vi "publish -- lorentzian.vi"(7 "publisher action":T3, 9 "lorentzian IN":T1={"A (VHz)"=1.0, "f (Hz)"=1000.0, "G (Hz)"=3.0, "phi(rad)"=0.0, "Q"=300.0, "Norm  Ampl"=nan, "bg (V)"=0.0+0.0i, "4corners"={"z (-pi/2)"=9.277908004825974e-07+0.0007240755403629966i, "z(inf)"=2.6527949823343002e-05+0.0007477540585896028i, "z (pi/2)"=2.8494315967368497e-06+0.0007733542176124632i, "z center"=1.8886111986097237e-06+0.0007487148789877299i, "z(0)"=-2.2750727426123552e-05+0.000749675699385857i, "radius"=2.4658065287076567e-05}} {"bg (V)" format="%#_3p"; "Q" format="%#_4p"; "phi(rad)" format="%#_3p"; "G (Hz)" format="%#_4p"; "f (Hz)" format="%#_6p"; "A (VHz)" format="%#_3p"}) -> (1 "lorentzian OUT":T1={"A (VHz)"=1.0, "f (Hz)"=1000.0, "G (Hz)"=3.0, "phi(rad)"=0.0, "Q"=300.0, "Norm  Ampl"=nan, "bg (V)"=0.0+0.0i, "4corners"={"z (-pi/2)"=9.277908004825974e-07+0.0007240755403629966i, "z(inf)"=2.6527949823343002e-05+0.0007477540585896028i, "z (pi/2)"=2.8494315967368497e-06+0.0007733542176124632i, "z center"=1.8886111986097237e-06+0.0007487148789877299i, "z(0)"=-2.2750727426123552e-05+0.000749675699385857i, "radius"=2.4658065287076567e-05}} {"bg (V)" format="%#_3p"; "Q" format="%#_4p"; "phi(rad)" format="%#_3p"; "G (Hz)" format="%#_4p"; "f (Hz)" format="%#_6p"; "A (VHz)" format="%#_3p"})   [LabVIEW 2020]
uses:
  publisher action.ctl
  lorentzian.ctl
  circle corners.ctl
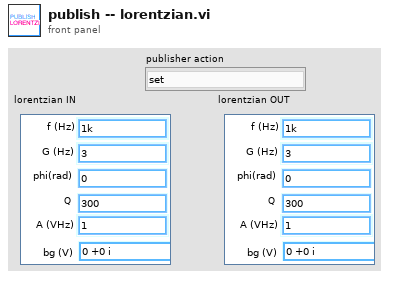
[diagram p1: front panel]
types:
  T1 = typedef "lorentzian.ctl" = cluster{"A (VHz)":dbl, "f (Hz)":dbl, "G (Hz)":dbl, "phi(rad)":dbl, "Q":dbl, "Norm  Ampl":dbl, "bg (V)":cdb, "4corners":T2}
  T2 = typedef "circle corners.ctl" = cluster{"z (-pi/2)":cdb, "z(inf)":cdb, "z (pi/2)":cdb, "z center":cdb, "z(0)":cdb, "radius":dbl}
  T3 = typedef "publisher action.ctl" = enum16{"set", "get", "init", "check"}
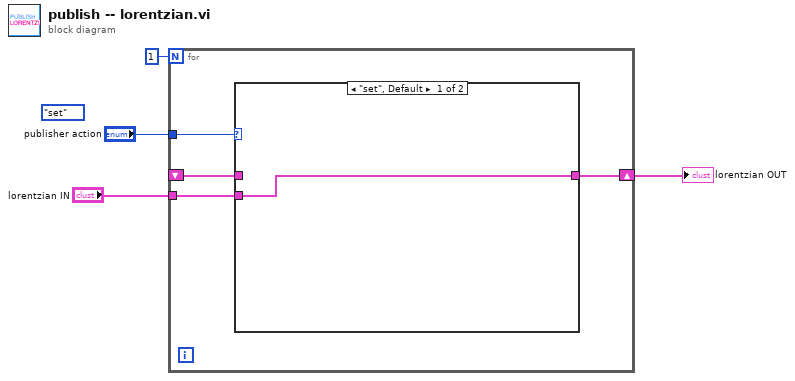
[diagram p0: block diagram]
diagram:
  (unwired) publisher_action."set" ("publisher action")
  n1 = for {
    N: 1 -> [_]
    tunnel: "publisher action" -> [w8]
    tunnel: "lorentzian IN" -> [w6]
    shift-right: [w7] -> w1
    shift-left: _ -> [w5]
    n2 = case shown="\"set\", Default" w8 {
      tunnel: [w9 w10] -> w7
      tunnel: w6 -> [w9 _]
      tunnel: w5 -> [_ w10]
      frame "set", Default {
      }
      frame "get" {
      }
    }
  }
  "lorentzian OUT" <- w1
